vi "SnapPhoto.vi"(8 "error in":errorcluster, 11 "Session In":T1="cam0") -> (0 "error out":errorcluster, 3 "Image Out":T2)   [LabVIEW 2019]
uses:
  <vilib>/vision/Image Controls.llb/IMAQ Image.ctl
  <vilib>/userDefined/High Color/IMAQdx.ctl
  <vilib>/vision/driver/NI_Vision_Acquisition_Software.lvlib
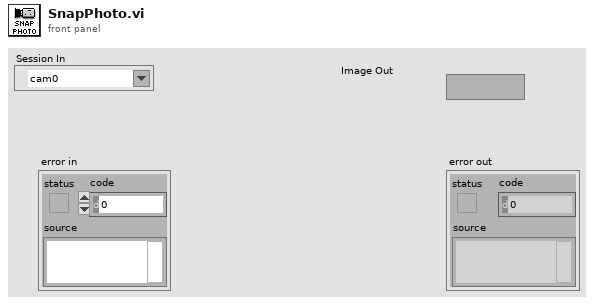
[diagram p1: front panel]
types:
  T1 = typedef "IMAQdx.ctl" = refnum<k21>
  T2 = typedef "IMAQ Image.ctl" = refnum<image>
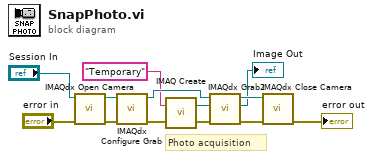
[diagram p0: block diagram]
diagram:
  # "Photo acquisition"
  n1 = call <vilib>:"IMAQdx Open Camera.vi"("error in"="error in", "Session In"="Session In") -> ("error out"=w13:errorcluster, "Session Out"=w12:T1)  [unwired: 8 in]
  n2 = call <vilib>:"IMAQdx Configure Grab.vi"("error in"=w13, "Session In"=w12) -> ("error out"=w2:errorcluster, "Session Out"=w11:T1)  [unwired: 8 in]
  n3 = call "IMAQ Create"("Image Name"="Temporary", "error in (no error)"=w2) -> ("New Image"=w7:T2, "error out"=w1:errorcluster)  [unwired: 3 in]
  n4 = call <vilib>:"IMAQdx Grab2.vi"("error in"=w1, "Image In"=w7, "Session In"=w11) -> ("error out"=w10:errorcluster, "Image Out"=→"Image Out":T2, "Session Out"=w9:T1)  [unwired: 5 in, 1 out]
  n5 = call <vilib>:"IMAQdx Close Camera.vi"("error in"=w10, "Session In"=w9) -> ("error out"=→"error out":errorcluster)  [unwired: 9 in]
